vi "EEV Position.vi"() -> (3 "DSM Message":string)   [LabVIEW 2014, in "GEA2_Toolkit.lvlib"]
uses:
  Labview GEA2 Toolkit v2.1/library/GEA2_Toolkit.lvlib
  Custom Pallet Controls/Forward.ctl
panel:
  in  "EEV Position":u16
  out "Description":string="Set EEV Position"
  in  "Complete":T1
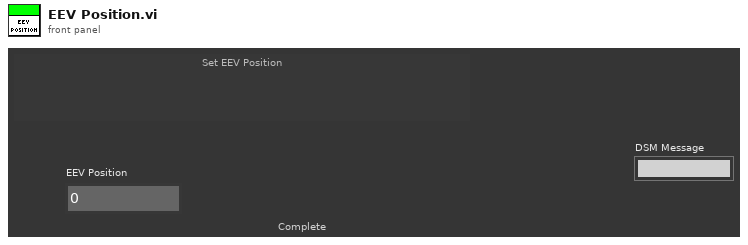
[diagram p1: front panel]
types:
  T1 = typedef "GEA2_Toolkit.lvlib/Forward.ctl" = bool
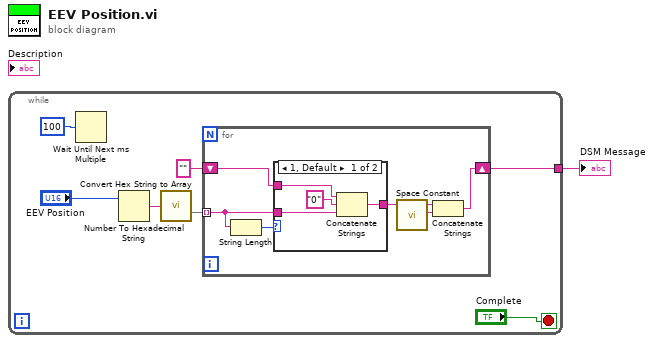
[diagram p0: block diagram]
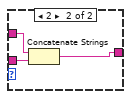
[diagram p2: hidden frame]
diagram:
  n1 = while {
    tunnel: [w2] -> w1
    stop <- "Complete" stop-if-true
    n2 = Wait Until Next ms Multiple(millisecond multiple=u32 100) -> ()  [unwired: 1 out]
    n3 = Number To Hexadecimal String(2:"EEV Position") -> (0:w5:string)  [unwired: 1 in]
    n4 = call "Convert Hex String to Array.vi"("Hex String In"=w5) -> (10:w4)  [unwired: 13 in, 1 out]
    n5 = for {
      tunnel: w4 -> [w12] mode=indexing
      shift-right: [w9] -> w2
      shift-left: "" -> [w13]
      n6 = String Length(string=w12) -> (length=w14:i32)
      n7 = case shown="1, Default" w14 {
        tunnel: w13 -> [w18 w21]
        tunnel: [w15 w20] -> w10
        tunnel: w12 -> [w16 w19]
        frame 1, Default {
          n8 = Concatenate Strings(w18, "0" ("string"), w16) -> (w15:string)
        }
        frame 2 {
          n9 = Concatenate Strings(w21, w19) -> (w20:string)
        }
      }
      n10 = call <vilib>:"Space Constant.vi"() -> ("String"=w11:string)
      n11 = Concatenate Strings(w10, w11) -> (w9:string)
    }
  }
  "DSM Message" <- w1
